vi "Untitled 1.vi"() -> ()   [LabVIEW 2017]
uses:
  <vilib>/measure/mamon.llb/Waveform Peak Detection for 1 Chan.vi
  <vilib>/measure/NI_MAPro.lvlib
panel:
  out "GHz/sec":dbl
  out "dt":dbl format="%#_4g"
  out "Locations":dbl[](array[numeric]) format="%.2p"
  out "Amplitudes":dbl[](array[numeric]) format="%.2p"
  out "2nd Derivatives":dbl[](array[numeric]) format="%.2p"
  out "Waveform Graph":dynamicdata(graph)
  in  "stop":bool
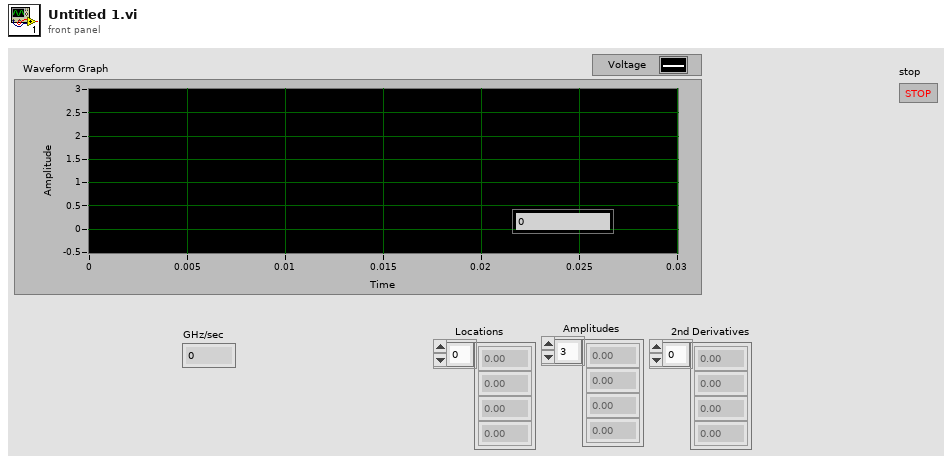
[diagram p1: front panel]
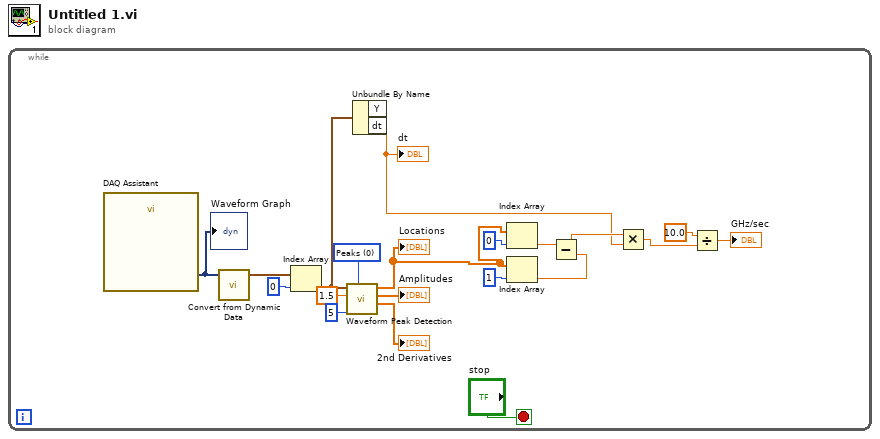
[diagram p0: block diagram]
diagram:
  n1 = while {
    stop <- "stop" stop-if-true
    w1 = u16 0 items=["Peaks", "Valleys"] ("peaks/valleys")
    n2 = call "DAQ Assistant"() -> ("data"=w17:dynamicdata)  [unwired: 17 in, 2 out]
    "Waveform Graph" <- w17
    n3 = call "Convert from Dynamic Data"("Dynamic Data Type"=w17) -> ("Array of Waveform"=w19:waveform(dbl)[])  [unwired: 3 in]
    n4 = Index Array(array=w19, index=0) -> (element=w12:waveform(dbl))
    n5 = call-poly <vilib>:"Waveform Peak Detection.vi"("peaks/valleys"=w1, "width"=5, "threshold"=1.5, "Signal In"=w12) -> ("2nd Derivatives"=→"2nd Derivatives":dbl[], "Amplitudes"=→"Amplitudes":dbl[], "Locations"=w11:dbl[])  [unwired: 3 in, 2 out]
    "Locations" <- w11
    n6 = Unbundle By Name(w12) -> ("dt"=w7:dbl)  [unwired: 1 out]
    "dt" <- w7
    n7 = Index Array(array=w11, index=0 ("length")) -> (element=w8:dbl)
    n8 = Index Array(array=w11, index=1) -> (element=w9:dbl)
    n9 = Subtract(x=w8, y=w9) -> (x-y=w10:dbl)
    n10 = Multiply(x=w10, y=w7) -> (x*y=w4:dbl)
    n11 = Divide(x=10.0, y=w4) -> (x/y=→"GHz/sec":dbl)
  }
